vi "Display Info.vi"(7 "Layout ref":refnum<vi>, 8 "error in (no error)":errorcluster, 9 "Modify (F) /Add [T]":bool, 10 "Names in use":string[](array[string]), 11 "SRS_SG380 in":refnum<class "SRS_SG380.lvclass">) -> (0 "error out":errorcluster, 1 "Names in use out":string[](array[string]), 2 "Changes Made?":bool, 3 "SRS_SG380 out":refnum<class "SRS_SG380.lvclass">)   [LabVIEW 2013, in "SRS_SG380.lvclass"]
uses:
  SRS_SG380.lvclass
  TypeDefs/ColumnAppearCluster.ctl
  SRS_SG380.lvclass/SRS_SG380.ctl
  ColumnVIs/Column/Column.lvclass
panel:
  in  "Amplitude Column Apperance":T1={"Column Name"="Amplitude", "Width"=30, "Bkgd"=[16448250], "Text"=[0]}
  in  "Freq Column Appearance":T1={"Column Name"="Frequency", "Width"=30, "Bkgd"=[16448250], "Text"=[0]}
  in  "Cancel":bool
  in  "Done":bool
  in  "Hardware Settings":T2={"PB Trigger Line"=65535, "Serial Port"=""}
  in  "Device Description":string
  in  "Name":string
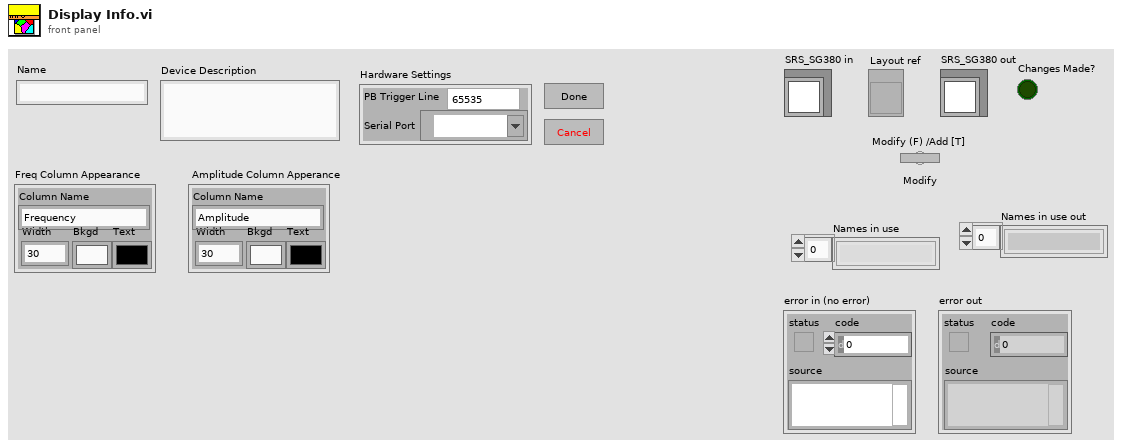
[diagram p1: front panel]
types:
  T1 = typedef "ColumnAppearCluster.ctl" = cluster{"Column Name":string, "Width":u32, "Bkgd":u32[], "Text":u32[]}
  T2 = cluster{"PB Trigger Line":u16, "Serial Port":refnum<visa-resource-name>}
  T3 = cluster{u16, "Serial Port":refnum<visa-resource-name>}
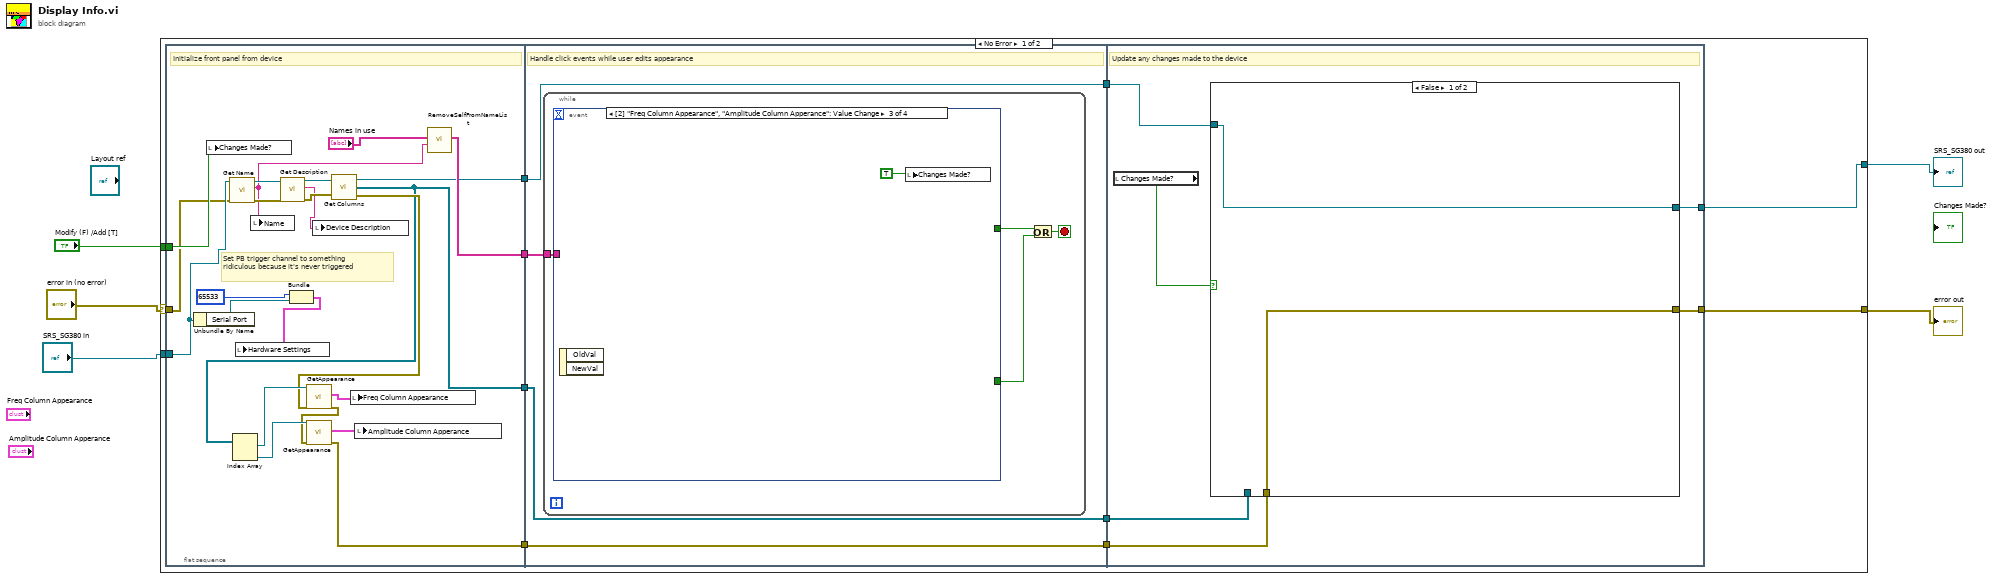
[diagram p0: block diagram]
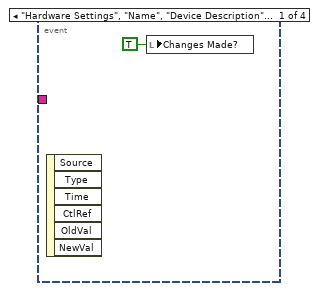
[diagram p2: hidden frame]
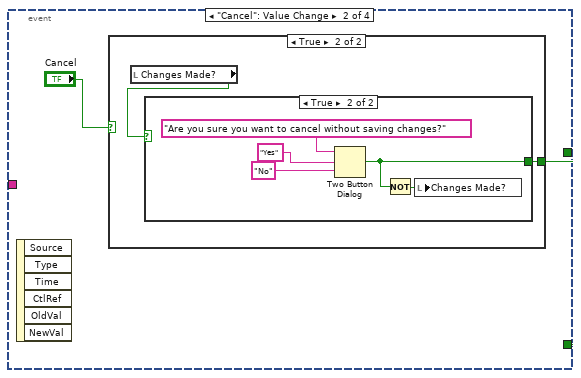
[diagram p3: hidden frame]
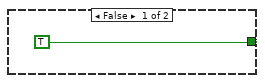
[diagram p5: hidden frame]
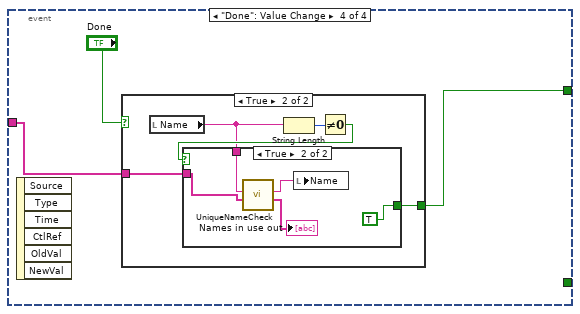
[diagram p6: hidden frame]
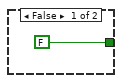
[diagram p7: hidden frame]
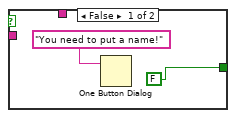
[diagram p8: hidden frame]
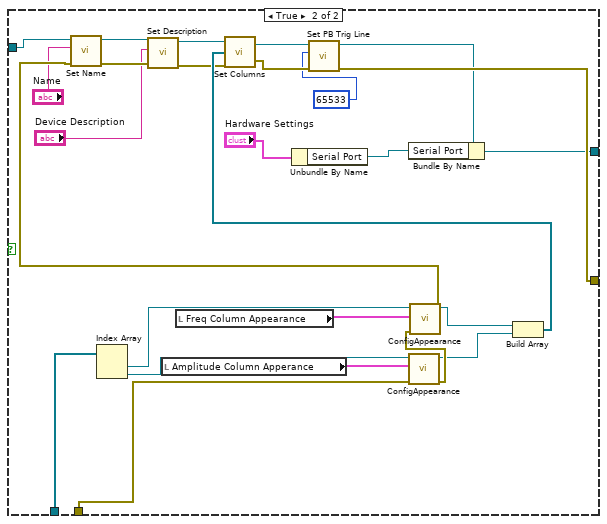
[diagram p9: hidden frame]
diagram:
  n1 = case shown="No Error" "error in (no error)" {
    selector: "error in (no error)" -> [w15 w113]
    tunnel: [w7 w113] -> w1
    tunnel: [w6 w112] -> w2
    tunnel: "SRS_SG380 in" -> [w16 w112]
    tunnel: "Modify (F) /Add [T]" -> [w17 _]
    frame No Error {
      n2 = flat-sequence {
        tunnel: w17 -> [w40]
        tunnel: w16 -> [w36]
        tunnel: w15 -> [w34]
        tunnel: [w22] -> w14
        tunnel: [w21] -> w13
        tunnel: [w20] -> w11
        tunnel: [w18] -> w9
        tunnel: w14 -> [w44]
        tunnel: w13 -> [w43]
        tunnel: [w43] -> w12
        tunnel: w11 -> [w42]
        tunnel: [w42] -> w10
        tunnel: w9 -> [w41]
        tunnel: [w41] -> w8
        tunnel: w12 -> [w83]
        tunnel: w10 -> [w82]
        tunnel: w8 -> [w81]
        tunnel: [w79] -> w7
        tunnel: [w78] -> w6
        frame #0 {
          # "Set PB trigger channel to something ridiculous because it's never triggered"
          # "Initialize front panel from device"
          n3 = Unbundle By Name(w36) -> ("Serial Port"=w38:refnum<visa-resource-name>)
          n4 = local write "Changes Made?"(w40) -> ()
          n5 = call-dynamic "Get Name.vi"("error in (no error)"=w34, "Device in"=w36) -> ("error out"=w33:errorcluster, "Name"=w30:string, "Device out"=w35:refnum<class "SRS_SG380.lvclass">)  [unwired: 7 in]
          n6 = local write "Name"(w30) -> ()
          n7 = call-dynamic "Get Description.vi"("error in (no error)"=w33, "Device in"=w35) -> ("error out"=w31:errorcluster, "Device Description"=w29:string, "Device out"=w32:refnum<class "SRS_SG380.lvclass">)  [unwired: 7 in]
          n8 = Bundle(u16 65533, "Serial Port"=w38) -> (w37:T3)  [unwired: 1 in]
          n9 = local write "Hardware Settings"(w37) -> ()
          n10 = local write "Device Description"(w29) -> ()
          n11 = call-dynamic "Get Columns.vi"("Device in"=w32, "error in (no error)"=w31) -> ("Device out"=w21:refnum<class "SRS_SG380.lvclass">, "Columns"=w20:refnum<class "Column.lvclass">[], "error out"=w26:errorcluster)
          n12 = Index Array(array=w20) -> (element #1=w28:refnum<class "Column.lvclass">, element #2=w27:refnum<class "Column.lvclass">)  [unwired: 2 in]
          n13 = call "GetAppearance.vi"("error in (no error)"=w26, "Column in"=w28) -> ("error out"=w25:errorcluster, "Column Appearance"=w24:T1)  [unwired: 7 in, 1 out]
          n14 = call "GetAppearance.vi"("error in (no error)"=w25, "Column in"=w27) -> ("error out"=w18:errorcluster, "Column Appearance"=w23:T1)  [unwired: 7 in, 1 out]
          n15 = local write "Freq Column Appearance"(w24) -> ()
          n16 = local write "Amplitude Column Apperance"(w23) -> ()
          n17 = call "RemoveSelfFromNameList.vi"("self Name"=w30, "Names in use"="Names in use") -> ("Reserved Names"=w22:string[])  [unwired: 9 in]
        }
        frame #1 {
          # "Handle click events while user edits appearance"
          n18 = while {
            tunnel: w44 -> [w45]
            stop <- w48 stop-if-true
            n19 = event shown="[2] \"Freq Column Appearance\", \"Amplitude Column Apperance\": Value Change" {
              selector: _ -> [_ _ _ _]
              dyn-events: _ -> [_ _ _ _]
              timeout: _ -> [_ _ _ _]
              tunnel: [_ w51 _ _] -> w47
              tunnel: [_ _ _ w64] -> w46
              tunnel: w45 -> [_ _ _ w63]
              event "Hardware Settings", "Name", "Device Description": Value Change {
                n20 = event-data() -> ()  [unwired: 1 in, 6 out]
                n21 = local write "Changes Made?"(TRUE ("Changes Made?")) -> ()
              }
              event "Cancel": Value Change {
                n22 = event-data() -> ()  [unwired: 1 in, 6 out]
                n23 = case shown="True" "Cancel" {
                  selector: "Cancel" -> [w52 _]
                  tunnel: [w52 w54] -> w51
                  frame False {
                  }
                  frame True {
                    n24 = local read "Changes Made?"() -> (w53:bool)
                    n25 = case shown="True" w53 {
                      tunnel: [TRUE w57] -> w54
                      frame False {
                      }
                      frame True {
                        n26 = Two Button Dialog(message="Are you sure you want to cancel without saving changes?", 1:"No", 2:"Yes") -> (T button?=w57:bool)
                        n27 = Not(x=w57) -> (.not. x?=w56:bool)
                        n28 = local write "Changes Made?"(w56) -> ()
                      }
                    }
                  }
                }
              }
              event Value Change {
                n29 = event-data() -> ()  [unwired: 1 in, 2 out]
                n30 = local write "Changes Made?"(TRUE) -> ()
              }
              event "Done": Value Change {
                n31 = event-data() -> ()  [unwired: 1 in, 6 out]
                n32 = case shown="True" "Done" {
                  tunnel: [FALSE w68] -> w64
                  tunnel: w63 -> [_ w67]
                  frame False {
                  }
                  frame True {
                    n33 = local read "Name"() -> (w66:string)
                    n34 = String Length(string=w66) -> (length=w70:i32)
                    n35 = Not Equal To 0?(x=w70) -> (x != 0?=w69:bool)
                    n36 = case shown="True" w69 {
                      tunnel: [FALSE TRUE] -> w68
                      tunnel: w67 -> [_ w76]
                      tunnel: w66 -> [_ w75]
                      frame False {
                        n37 = One Button Dialog(message="You need to put a name!") -> ()  [unwired: 1 in, 1 out]
                      }
                      frame True {
                        n38 = call "UniqueNameCheck.vi"("Names in use"=w76, "Device Name"=w75) -> ("Names in use out"=→"Names in use out":string[], "Unique name"=w74:string)  [unwired: 8 in]
                        n39 = local write "Name"(w74) -> ()
                      }
                    }
                  }
                }
              }
            }
            n40 = Or(x=w46, y=w47) -> (x .or. y?=w48:bool)
          }
        }
        frame #2 {
          # "Update any changes made to the device"
          n41 = local read "Changes Made?"() -> (w80:bool)
          n42 = case shown="False" w80 {
            tunnel: w83 -> [w85 w111]
            tunnel: w82 -> [_ w109]
            tunnel: w81 -> [w84 w86]
            tunnel: [w84 w94] -> w79
            tunnel: [w85 w91] -> w78
            frame False {
            }
            frame True {
              n43 = Index Array(array=w109) -> (element #1=w108:refnum<class "Column.lvclass">, element #2=w107:refnum<class "Column.lvclass">)  [unwired: 2 in]
              n44 = local read "Amplitude Column Apperance"() -> (w102:T1)
              n45 = local read "Freq Column Appearance"() -> (w103:T1)
              n46 = Unbundle By Name("Hardware Settings") -> ("Serial Port"=w92:refnum<visa-resource-name>)
              n47 = call "ConfigAppearance.vi"("error in (no error)"=w86, "Column Appearance"=w102, "Column in"=w107) -> ("error out"=w106:errorcluster, "Column out"=w100:refnum<class "Column.lvclass">)  [unwired: 7 in]
              n48 = call "ConfigAppearance.vi"("error in (no error)"=w106, "Column Appearance"=w103, "Column in"=w108) -> ("error out"=w105:errorcluster, "Column out"=w101:refnum<class "Column.lvclass">)  [unwired: 7 in]
              n49 = call-dynamic "Set Name.vi"("error in (no error)"=w105, "Name"="Name", "Device in"=w111) -> ("error out"=w104:errorcluster, "Device out"=w110:refnum<class "SRS_SG380.lvclass">)  [unwired: 7 in]
              n50 = call-dynamic "Set Description.vi"("error in (no error)"=w104, "Device Description"="Device Description", "Device in"=w110) -> ("error out"=w97:errorcluster, "Device out"=w98:refnum<class "SRS_SG380.lvclass">)  [unwired: 7 in]
              n51 = Build Array(w101, w100) -> (w99:refnum<class "Column.lvclass">[])
              n52 = call-dynamic "Set Columns.vi"("error in (no error)"=w97, "Columns"=w99, "Device in"=w98) -> ("error out"=w95:errorcluster, "Device out"=w96:refnum<class "SRS_SG380.lvclass">)  [unwired: 1 in]
              n53 = call-dynamic "Set PB Trig Line.vi"("error in (no error)"=w95, "PB Trigger Line"=u16 65533, "Device in"=w96) -> ("error out"=w94:errorcluster, "Device out"=w93:refnum<class "SRS_SG380.lvclass">)  [unwired: 7 in]
              n54 = Bundle By Name(cluster=w93, "Serial Port"=w92) -> (w91:refnum<class "SRS_SG380.lvclass">)
            }
          }
        }
      }
    }
    frame Error {
    }
  }
  "error out" <- w1
  "SRS_SG380 out" <- w2
